vi "subscribed name change.vi"(8 "error in (no error)":errorcluster, 10 "top array":T1[](array[typedef]), 11 "BluePlotHandle":refnum<class "RocketPlotHandle.lvclass">) -> (0 "error out":errorcluster)   [LabVIEW 2021, in "RocketPlot.lvlib"]
uses:
  RocketPlot.lvlib
  Classes/RocketPlotHandle/RocketPlotHandle.lvclass
  TypeDefs/Plot top row.ctl
  <userlib>/_OpenG.lib/array/array.llb/Remove Duplicates from 1D Array (String)__ogtk.vi
  <userlib>/_OpenG.lib/array/array.llb/openg_array.lvlib
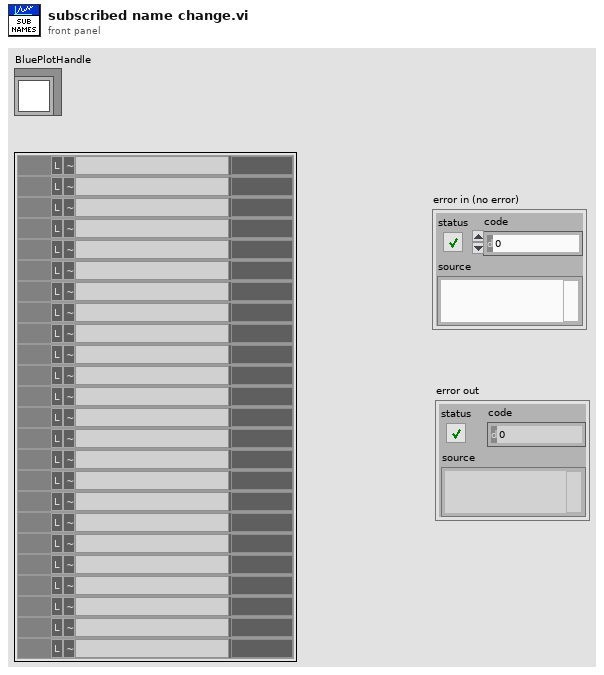
[diagram p1: front panel]
types:
  T1 = typedef "RocketPlot.lvlib/Plot top row.ctl" = cluster{"PID":string, "index":i32, "PID color":u32, "right axis?":bool, "Flatline?":bool, "Numeric color":u32, "Data":string, "Flat":string}
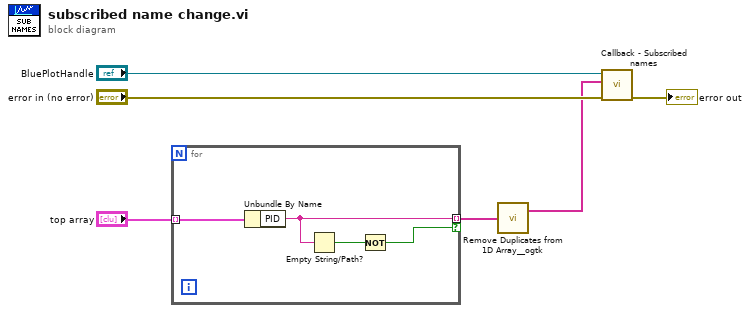
[diagram p0: block diagram]
diagram:
  n1 = for {
    tunnel: "top array" -> [w10] mode=indexing
    tunnel: [w9] -> w2 mode=indexing if=w7
    n2 = Unbundle By Name(w10) -> ("PID"=w9:string)
    n3 = Empty String/Path?(string/path=w9) -> (empty?=w8:bool)
    n4 = Not(x=w8) -> (.not. x?=w7:bool)
  }
  n5 = call-poly <userlib>:"Remove Duplicates from 1D Array__ogtk.vi"("Input Array"=w2) -> ("Output Array"=w1:string[])  [unwired: 1 out]
  n6 = call-dynamic "Callback - Subscribed names.vi"("error in (no error)"="error in (no error)", "Subscribed names"=w1, "BluePlotHandle in"="BluePlotHandle") -> ("error out"=→"error out":errorcluster)  [unwired: 7 in, 1 out]
